vi "SPI.Get Alice ID.vi"() -> (3 "Alice.ID":u8=2)   [LabVIEW 2018]
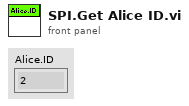
[diagram p1: front panel]
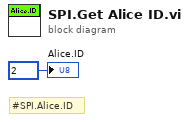
[diagram p0: block diagram]
diagram:
  # "#SPI.Alice.ID"
  "Alice.ID" <- u8 2
